vi "InitDataSets.vi"(8 "error in (no error)":errorcluster, 10 "registry":T3, 11 "dataevent":T1) -> (0 "error out":errorcluster, 2 "datasetIds":variant, 3 "datasets":T7[](array[typedef]))   [LabVIEW 2017, in "DataEventCreator.lvlib"]
uses:
  <vilib>/addons/InsightCM/Devices/Shared/Common/DataEventCreator/DataEventCreator.lvlib
  <vilib>/addons/InsightCM/Devices/Shared/Common/DataEvent/controls/DataSet.ctl
  <vilib>/addons/InsightCM/MessageBus/Base/controls/DataSetMetadata.ctl
  <vilib>/addons/InsightCM/MessageBus/Base/controls/KeyValuePair.ctl
  <vilib>/addons/InsightCM/Devices/Shared/Cms/CmsDataEventCreator/controls/GroupRegistry.ctl
  <vilib>/addons/InsightCM/Devices/Shared/Cms/CmsDataEventCreator/controls/DataSetRegistry.ctl
  <vilib>/addons/InsightCM/Devices/Shared/Common/DataEvent/controls/DataSetType.ctl
  <vilib>/addons/InsightCM/Devices/Shared/Common/DataEventCreator/controls/Registry_Trend.ctl
  <vilib>/addons/InsightCM/MessageBus/Base/controls/DataEvent.ctl
  <vilib>/addons/InsightCM/Devices/Shared/Common/DataEvent/DataEvent.lvlib
  <vilib>/addons/InsightCM/SRP/SRP.lvlib
  <vilib>/addons/InsightCM/Utilities/PropertyHelpers/PropertyHelpers.lvlib
  <vilib>/addons/InsightCM/Devices/Shared/Cms/CmsDataEventCreator/CmsDataEventCreator.lvlib
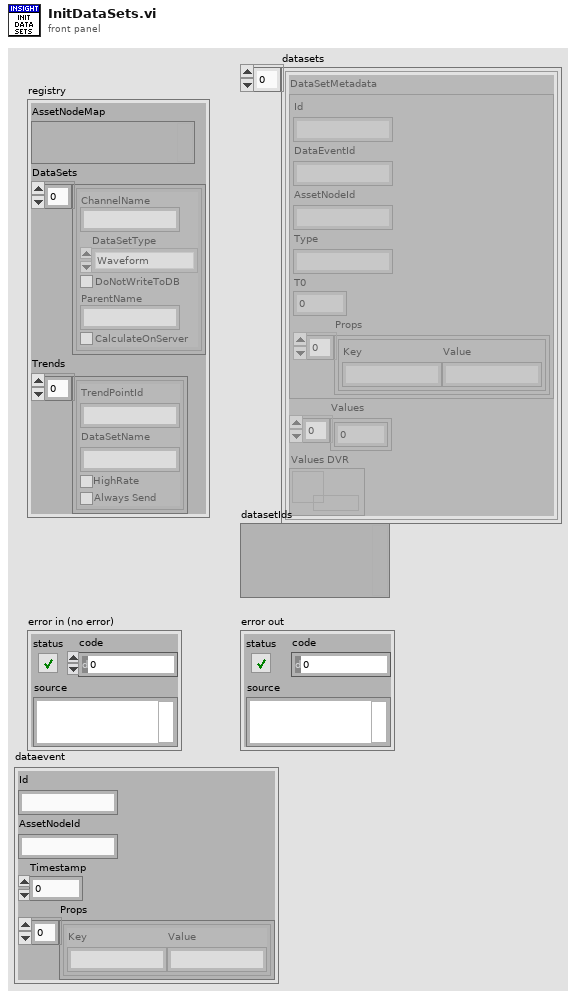
[diagram p1: front panel]
types:
  T1 = typedef "DataEvent.ctl" = cluster{"Id":string, "AssetNodeId":string, "Timestamp":i64, "Props":T2[]}
  T2 = typedef "KeyValuePair.ctl" = cluster{"Key":string, "Value":string}
  T3 = typedef "CmsDataEventCreator.lvlib/GroupRegistry.ctl" = cluster{"AssetNodeMap":variant, "DataSets":T4[], "Trends":T6[]}
  T4 = typedef "CmsDataEventCreator.lvlib/DataSetRegistry.ctl" = cluster{"ChannelName":string, "DataSetType":T5, "DoNotWriteToDB":bool, "ParentName":string, "CalculateOnServer":bool}
  T5 = typedef "DataEvent.lvlib/DataSetType.ctl" = enum16{"Waveform", "SpeedProfile", "ThermalImage", "EmsaSweep"}
  T6 = typedef "DataEventCreator.lvlib/Registry_Trend.ctl" = cluster{"TrendPointId":string, "DataSetName":string, "HighRate":bool, "Always Send":bool}
  T7 = typedef "DataEvent.lvlib/DataSet.ctl" = cluster{"DataSetMetadata":T8, "Values":sgl[], "Values DVR":refnum<data-value>}
  T8 = typedef "DataSetMetadata.ctl" = cluster{"Id":string, "DataEventId":string, "AssetNodeId":string, "Type":string, "T0":i64, "Props":T2[]}
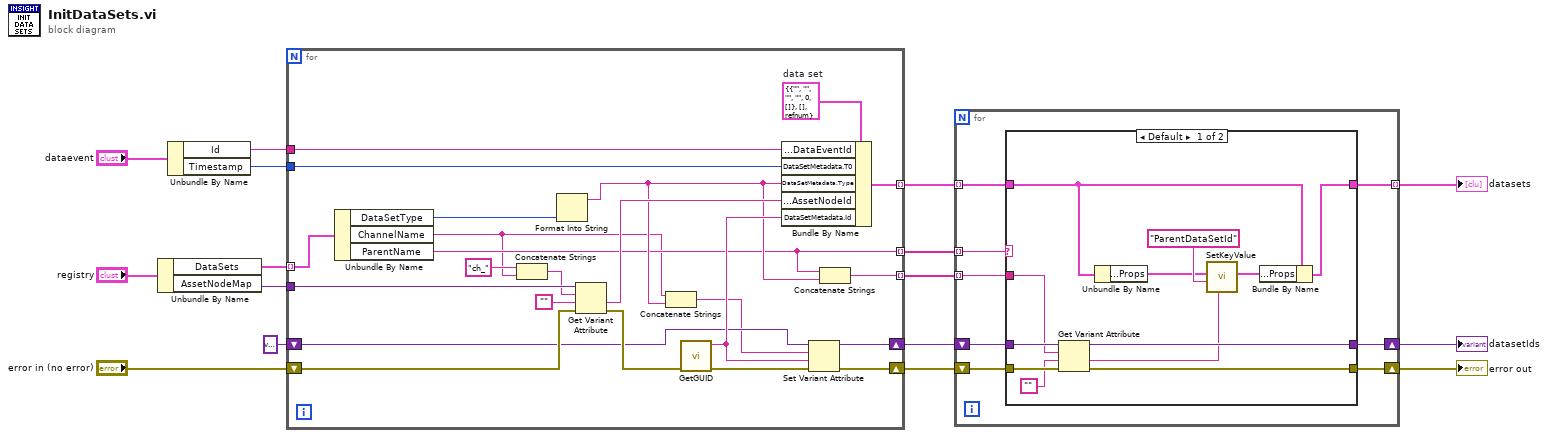
[diagram p0: block diagram]
diagram:
  n1 = Unbundle By Name("registry") -> ("DataSets"=w6:T4[], "AssetNodeMap"=w8:variant)
  n2 = Unbundle By Name("dataevent") -> ("Id"=w3:string, "Timestamp"=w2:i64)
  n3 = for {
    tunnel: w6 -> [w27] mode=indexing
    tunnel: w8 -> [w33]
    shift-right: [w38] -> w11
    shift-left: variant -> [w26]
    shift-right: [w37] -> w12
    shift-left: "error in (no error)" -> [w35]
    tunnel: [w29] -> w10 mode=indexing
    tunnel: [w22] -> w15 mode=indexing
    tunnel: w3 -> [w25]
    tunnel: w2 -> [w24]
    tunnel: [w20] -> w1 mode=indexing
    w31 = T7 {"DataSetMetadata"={"Id"="", "DataEventId"="", "AssetNodeId"="", "Type"="", "T0"=0, "Props"=[]}, "Values"=[], "Values DVR"=refnum}  # data set
    n4 = Unbundle By Name(w27) -> ("DataSetType"=w36:T5, "ChannelName"=w18:string, "ParentName"=w20:string)
    n5 = Concatenate Strings("ch_" ("string"), w18) -> (w17:string)
    n6 = Format Into String(w36) -> (resulting string=w21:string)  [unwired: 3 in, 1 out]
    n7 = Get Variant Attribute(Variant=w33, name=w17, default value (empty Variant)="", error in=w35) -> (value=w30:string, error out=w34:errorcluster)  [unwired: 2 out]
    n8 = Concatenate Strings(w18, w21) -> (w23:string)
    n9 = call <vilib>:"GetGUID.vi"("error in (no error)"=w34) -> ("error out"=w39:errorcluster, "GUID"=w28:string)  [unwired: 9 in]
    n10 = Bundle By Name(cluster=w31, "DataSetMetadata.DataEventId"=w25, "DataSetMetadata.T0"=w24, "DataSetMetadata.Type"=w21, "DataSetMetadata.AssetNodeId"=w30, "DataSetMetadata.Id"=w28) -> (w29:T7)
    n11 = Set Variant Attribute(Variant=w26, name=w23, value=w28, error in=w39) -> (Variant out=w38:variant, error out=w37:errorcluster)  [unwired: 1 out]
    n12 = Concatenate Strings(w20, w21) -> (w22:string)
  }
  n13 = for {
    tunnel: w10 -> [w47] mode=indexing
    shift-right: [w44] -> w13
    shift-left: w11 -> [w46]
    shift-right: [w43] -> w14
    shift-left: w12 -> [w45]
    tunnel: w15 -> [w41] mode=indexing
    tunnel: [w42] -> w16 mode=indexing
    tunnel: w1 -> [w40] mode=indexing
    n14 = case shown="Default" w40 {
      tunnel: w47 -> [w49 w60]
      tunnel: w46 -> [w59 w62]
      tunnel: w45 -> [w58 w61]
      tunnel: [w55 w62] -> w44
      tunnel: [w54 w61] -> w43
      tunnel: [w51 w60] -> w42
      tunnel: w41 -> [w50 _]
      frame Default {
        n15 = Get Variant Attribute(Variant=w59, name=w50, default value (empty Variant)="", error in=w58) -> (duplicate Variant=w55:variant, value=w53:string, error out=w54:errorcluster)  [unwired: 1 out]
        n16 = Unbundle By Name(w49) -> ("DataSetMetadata.Props"=w48:T2[])
        n17 = call <vilib>:"SetKeyValue.vi"("value"=w53, "key"="ParentDataSetId", "key value pairs"=w48) -> ("key value pairs out"=w56:T2[])  [unwired: 8 in]
        n18 = Bundle By Name(cluster=w49, "DataSetMetadata.Props"=w56) -> (w51:T7)
      }
      frame "" {
      }
    }
  }
  "datasets" <- w16
  "error out" <- w14
  "datasetIds" <- w13
